vi "Position Joystick Button.vi"(8 "error in (no error)":errorcluster, 11 "Button Ref":refnum<vi>) -> (0 "error out":errorcluster)   [LabVIEW 2014]
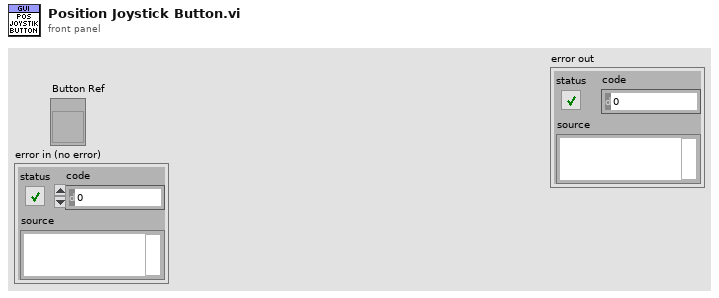
[diagram p1: front panel]
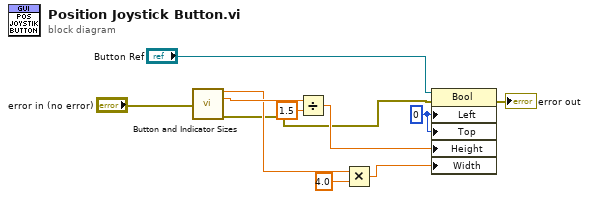
[diagram p0: block diagram]
diagram:
  w9 = 0 ("Position:Left")
  n1 = call "Button and Indicator Sizes.vi"("error in (no error)"="error in (no error)") -> ("Button Width"=w5:dbl, "Button Height"=w8:dbl, "error out"=w2:errorcluster)  [unwired: 10 in, 2 out]
  n2 = Divide(x=w8, y=1.5) -> (x/y=w6:dbl)
  n3 = Multiply(x=w5, y=4.0) -> (x*y=w3:dbl)
  n4 = property class="Bool"(reference="Button Ref", error in=w2, "Left"=w9, "Top"=w9, "Height"=w6, "Width"=w3) -> (error out=→"error out":errorcluster)  [unwired: 1 out]
